vi "Untitled 1.vi"() -> ()   [LabVIEW 2019]
uses:
  <vilib>/rvi/Emulation/niFpgaGetClockAttributes.vi
  <vilib>/rvi/Emulation/niFpgaSctlEmulationGetInTimedLoop.vi
  <vilib>/rvi/Emulation/niFpgaEmulationReportErrorSimple.vi
  <vilib>/rvi/eio/common/nirviEmuTemplateMethod_errors.vi
  <vilib>/rvi/Emulation/niFpgaCriticalErrorInLSC.vi
  <vilib>/eio/EIONode/EIONode.xnode
  <vilib>/eio/EIOMethodNode/EIOMethodNode.xnode
panel:
  out "number":u8
  in  "Enum":enum16{"z", "who am i", "y"}(ring)
  in  "stop":bool
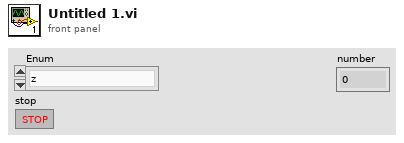
[diagram p1: front panel]
diagram:
  n1 = while {
    stop <- "stop" stop-if-true
    # "true =accelerometor"
    # "sou vi pour convertir binare to decimal"
    n2 = flat-sequence {
      tunnel: w1 -> [w16]
      tunnel: w6 -> [w30]
      tunnel: [w67] -> w2
      frame #0 {
        # "scl"
        # "sda ecriture"
        # "START CONDITION"
        n3 = xnode "FPGA I/O Node"("SDA"=TRUE ("ConnectorA/DIO9")) -> ()  [unwired: 1 in, 1 out]
        n4 = xnode "FPGA I/O Node"("SCL"=TRUE ("ConnectorA/DIO10")) -> ()  [unwired: 1 in, 1 out]
      }
      frame #1 {
        n5 = call "Wait"("Count(Ticks)"=u32 1000) -> ()  [unwired: 1 out]
      }
      frame #2 {
        # "sda ecriture"
        n6 = xnode "FPGA I/O Node"("SDA"=FALSE ("ConnectorA/DIO9")) -> ()  [unwired: 1 in, 1 out]
      }
      frame #3 {
        n7 = call "Wait2"("Count(Ticks)"=u32 1000) -> ()  [unwired: 1 out]
      }
      frame #4 {
        # "scl"
        n8 = xnode "FPGA I/O Node"("SCL"=FALSE ("ConnectorA/DIO10")) -> ()  [unwired: 1 in, 1 out]
      }
      frame #5 {
        # "on envoie l address du module voule accelerometre ou magnetic sensor"
        n9 = Number To Boolean Array(number=w16) -> (Boolean array=w15:bool[])
        n10 = Reverse 1D Array(array=w15) -> (reversed array=w14:bool[])
        n11 = for {
          tunnel: w14 -> [w17] mode=indexing
          n12 = flat-sequence {
            tunnel: w17 -> [w18]
            frame #0 {
              # "sda ecriture"
              n13 = xnode "FPGA I/O Node"("SDA"=w18) -> ()  [unwired: 1 in, 1 out]
            }
            frame #1 {
              n14 = call "Wait3"("Count(Ticks)"=u32 1000) -> ()  [unwired: 1 out]
            }
            frame #2 {
              # "scl"
              n15 = xnode "FPGA I/O Node"("SCL"=TRUE) -> ()  [unwired: 1 in, 1 out]
            }
            frame #3 {
              n16 = call "Wait10"("Count(Ticks)"=u32 1000) -> ()  [unwired: 1 out]
            }
            frame #4 {
              # "scl"
              n17 = xnode "FPGA I/O Node"("SCL"=FALSE) -> ()  [unwired: 1 in, 1 out]
            }
          }
        }
      }
      frame #6 {
        # "verifie s il"
        # "acknowledge slave"
        n18 = xnode "FPGA I/O Method Node"("Enable"=FALSE) -> ()  [unwired: 1 in, 1 out]
      }
      frame #7 {
        n19 = call "Wait4"("Count(Ticks)"=u32 1000) -> ()  [unwired: 1 out]
      }
      frame #8 {
        # "scl"
        n20 = xnode "FPGA I/O Node"("SCL"=TRUE) -> ()  [unwired: 1 in, 1 out]
      }
      frame #9 {
        n21 = call "Wait9"("Count(Ticks)"=u32 1000) -> ()  [unwired: 1 out]
      }
      frame #10 {
        # "scl"
        n22 = xnode "FPGA I/O Node"("SCL"=FALSE) -> ()  [unwired: 1 in, 1 out]
      }
      frame #11 {
        # "ecriture de l address du registre"
        # "il faut choisir la longeur de la donne avec deux on a le standrard CTRL_REG1_A"
        # "on doit envoyer l address du registre le standard c"
        n23 = Number To Boolean Array(number=w30) -> (Boolean array=w29:bool[])
        n24 = Reverse 1D Array(array=w29) -> (reversed array=w28:bool[])
        n25 = for {
          tunnel: w28 -> [w31] mode=indexing
          n26 = flat-sequence {
            tunnel: w31 -> [w32]
            frame #0 {
              # "sda ecriture"
              n27 = xnode "FPGA I/O Node"("SDA"=w32) -> ()  [unwired: 1 in, 1 out]
            }
            frame #1 {
              n28 = call "Wait8"("Count(Ticks)"=u32 1000) -> ()  [unwired: 1 out]
            }
            frame #2 {
              # "scl"
              n29 = xnode "FPGA I/O Node"("SCL"=TRUE) -> ()  [unwired: 1 in, 1 out]
            }
            frame #3 {
              n30 = call "Wait6"("Count(Ticks)"=u32 1000) -> ()  [unwired: 1 out]
            }
            frame #4 {
              # "scl"
              n31 = xnode "FPGA I/O Node"("SCL"=FALSE) -> ()  [unwired: 1 in, 1 out]
            }
          }
        }
      }
      frame #12 {
        # "acknowledge"
        n32 = flat-sequence {
          frame #0 {
            # "verifie s il"
            # "acknowledge slave"
            n33 = xnode "FPGA I/O Method Node"("Enable"=FALSE) -> ()  [unwired: 1 in, 1 out]
          }
          frame #1 {
            n34 = call "Wait23"("Count(Ticks)"=u32 1000) -> ()  [unwired: 1 out]
          }
          frame #2 {
            n35 = xnode "FPGA I/O Node"("SCL"=TRUE) -> ()  [unwired: 1 in, 1 out]
          }
          frame #3 {
            n36 = call "Wait24"("Count(Ticks)"=u32 1000) -> ()  [unwired: 1 out]
          }
          frame #4 {
            n37 = xnode "FPGA I/O Node"("SCL"=FALSE) -> ()  [unwired: 1 in, 1 out]
          }
        }
      }
      frame #13 {
        # "stop"
        n38 = flat-sequence {
          frame #0 {
            n39 = xnode "FPGA I/O Node"("SDA"=FALSE ("ConnectorA/DIO9")) -> ()  [unwired: 1 in, 1 out]
          }
          frame #1 {
            n40 = call "Wait11"("Count(Ticks)"=u32 1000 ("Tick Count(Ticks)")) -> ()  [unwired: 1 out]
          }
          frame #2 {
            n41 = xnode "FPGA I/O Node"("SDA"=TRUE ("ConnectorA/DIO9")) -> ()  [unwired: 1 in, 1 out]
          }
          frame #3 {
            n42 = call "Wait12"("Count(Ticks)"=u32 1000) -> ()  [unwired: 1 out]
          }
          frame #4 {
            n43 = xnode "FPGA I/O Node"("SCL"=TRUE) -> ()  [unwired: 1 in, 1 out]
          }
        }
      }
      frame #14 {
        # "start"
        n44 = flat-sequence {
          frame #0 {
            # "scl"
            # "sda ecriture"
            # "START CONDITION"
            n45 = xnode "FPGA I/O Node"("SDA"=TRUE ("ConnectorA/DIO9")) -> ()  [unwired: 1 in, 1 out]
            n46 = xnode "FPGA I/O Node"("SCL"=TRUE ("ConnectorA/DIO10")) -> ()  [unwired: 1 in, 1 out]
          }
          frame #1 {
            n47 = call "Wait19"("Count(Ticks)"=u32 1000) -> ()  [unwired: 1 out]
          }
          frame #2 {
            # "sda ecriture"
            n48 = xnode "FPGA I/O Node"("SDA"=FALSE ("ConnectorA/DIO9")) -> ()  [unwired: 1 in, 1 out]
          }
          frame #3 {
            n49 = call "Wait20"("Count(Ticks)"=u32 1000) -> ()  [unwired: 1 out]
          }
        }
      }
      frame #15 {
        # "on envoie l address du module voule accelerometre ou magnetic sensor"
        n50 = Number To Boolean Array(number=i8 50) -> (Boolean array=w54:bool[])
        n51 = Reverse 1D Array(array=w54) -> (reversed array=w53:bool[])
        n52 = for {
          tunnel: w53 -> [w55] mode=indexing
          n53 = flat-sequence {
            tunnel: w55 -> [w56]
            frame #0 {
              # "sda ecriture"
              n54 = xnode "FPGA I/O Node"("SDA"=w56) -> ()  [unwired: 1 in, 1 out]
            }
            frame #1 {
              n55 = call "Wait22"("Count(Ticks)"=u32 1000) -> ()  [unwired: 1 out]
            }
            frame #2 {
              # "scl"
              n56 = xnode "FPGA I/O Node"("SCL"=TRUE) -> ()  [unwired: 1 in, 1 out]
            }
            frame #3 {
              n57 = call "Wait21"("Count(Ticks)"=u32 1000) -> ()  [unwired: 1 out]
            }
            frame #4 {
              # "scl"
              n58 = xnode "FPGA I/O Node"("SCL"=FALSE) -> ()  [unwired: 1 in, 1 out]
            }
          }
        }
      }
      frame #16 {
        # "acknowledge"
        n59 = flat-sequence {
          frame #0 {
            # "verifie s il"
            # "acknowledge slave"
            n60 = xnode "FPGA I/O Method Node"("Enable"=FALSE) -> ()  [unwired: 1 in, 1 out]
          }
          frame #1 {
            n61 = call "Wait25"("Count(Ticks)"=u32 1000) -> ()  [unwired: 1 out]
          }
          frame #2 {
            n62 = xnode "FPGA I/O Node"("SCL"=TRUE) -> ()  [unwired: 1 in, 1 out]
          }
          frame #3 {
            n63 = call "Wait26"("Count(Ticks)"=u32 1000) -> ()  [unwired: 1 out]
          }
          frame #4 {
            n64 = xnode "FPGA I/O Node"("SCL"=FALSE) -> ()  [unwired: 1 in, 1 out]
          }
        }
      }
      frame #17 {
        # "important avant de lire a chaque fois"
        n65 = xnode "FPGA I/O Method Node"("Enable"=FALSE) -> ()  [unwired: 1 in, 1 out]
      }
      frame #18 {
        # "ca envoie 8 bit"
        n66 = for {
          N: 8 -> [_]
          tunnel: [w70] -> w68 mode=indexing
          n67 = flat-sequence {
            tunnel: [w71] -> w70
            frame #0 {
              # "sda lecture"
              n68 = xnode "FPGA I/O Node"() -> ("SDA"=w71:bool)  [unwired: 1 in, 1 out]
            }
            frame #1 {
              n69 = call "Wait5"("Count(Ticks)"=u32 1000) -> ()  [unwired: 1 out]
            }
            frame #2 {
              # "scl"
              n70 = xnode "FPGA I/O Node"("SCL"=TRUE) -> ()  [unwired: 1 in, 1 out]
            }
            frame #3 {
              n71 = call "Wait7"("Count(Ticks)"=u32 1000) -> ()  [unwired: 1 out]
            }
            frame #4 {
              # "scl"
              n72 = xnode "FPGA I/O Node"("SCL"=FALSE) -> ()  [unwired: 1 in, 1 out]
            }
          }
        }
        n73 = Reverse 1D Array(array=w68) -> (reversed array=w67:bool[])
      }
      frame #19 {
        # "nak by master"
        n74 = flat-sequence {
          frame #0 {
            n75 = xnode "FPGA I/O Node"("SDA"=TRUE ("ConnectorA/DIO9")) -> ()  [unwired: 1 in, 1 out]
          }
          frame #1 {
            n76 = call "Wait15"("Count(Ticks)"=u32 1000 ("Tick Count(Ticks)")) -> ()  [unwired: 1 out]
          }
          frame #2 {
            n77 = xnode "FPGA I/O Node"("SCL"=TRUE) -> ()  [unwired: 1 in, 1 out]
          }
          frame #3 {
            n78 = call "Wait16"("Count(Ticks)"=u32 1000 ("Tick Count(Ticks)")) -> ()  [unwired: 1 out]
          }
          frame #4 {
            n79 = xnode "FPGA I/O Node"("SCL"=FALSE) -> ()  [unwired: 1 in, 1 out]
          }
        }
      }
      frame #20 {
        # "stop"
        n80 = flat-sequence {
          frame #0 {
            n81 = xnode "FPGA I/O Node"("SDA"=FALSE ("ConnectorA/DIO9")) -> ()  [unwired: 1 in, 1 out]
          }
          frame #1 {
            n82 = call "Wait17"("Count(Ticks)"=u32 1000 ("Tick Count(Ticks)")) -> ()  [unwired: 1 out]
          }
          frame #2 {
            n83 = xnode "FPGA I/O Node"("SDA"=TRUE ("ConnectorA/DIO9")) -> ()  [unwired: 1 in, 1 out]
          }
          frame #3 {
            n84 = call "Wait18"("Count(Ticks)"=u32 1000) -> ()  [unwired: 1 out]
          }
          frame #4 {
            n85 = xnode "FPGA I/O Node"("SCL"=TRUE) -> ()  [unwired: 1 in, 1 out]
          }
        }
      }
    }
    n86 = call "selectionen accelerometre etmagneticsensrnsor.vi"("Boolean"=TRUE) -> ("address"=w1:i8)  [unwired: 10 in]
    n87 = call "selectionneur d axe de l accelerometre.vi"("Enum"="Enum") -> ("VALEUR NUMERIQUE DE L AXE CHOISI"=w6:i8)  [unwired: 10 in]
    n88 = Boolean Array To Number(Boolean array=w2) -> (number=→"number":u8)
  }
